vi "Generate Log Data.vi"(8 "error in (no error)":errorcluster, 11 "TestRec":T1) -> (0 "error out":errorcluster, 3 "Log Data":string[][](array[string]), 5 "CsvPath":path)   [LabVIEW 2011]
uses:
  Controls/DVR of CSV Tests Data.ctl
  Controls/CSVs Tests Data.ctl
  Controls/Test Column Data.ctl
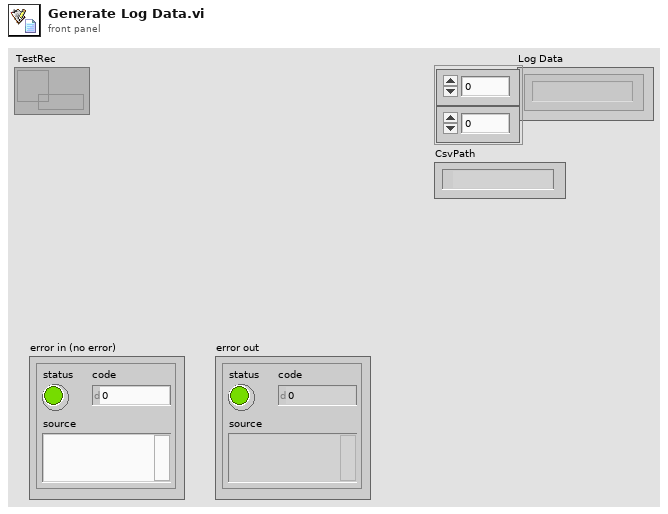
[diagram p1: front panel]
types:
  T1 = typedef "DVR of CSV Tests Data.ctl" = refnum<data-value>
  T2 = typedef "CSVs Tests Data.ctl" = cluster{"Test Data":T3[], "CsvPath":path, "LogPath":path, "Pass?":bool, "Error":errorcluster}
  T3 = typedef "Test Column Data.ctl" = cluster{"Chn":string, "ExpVals":dbl[], "TimeStamps":i64[], "NegTol":dbl, "PosTol":dbl}
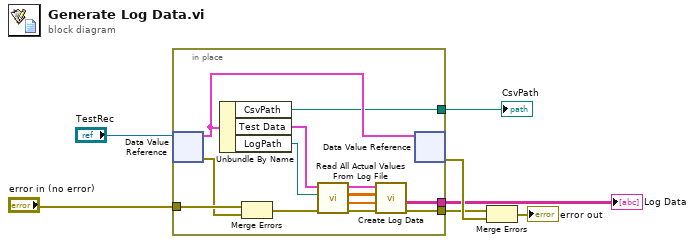
[diagram p0: block diagram]
diagram:
  n1 = in-place {
    in-place-border: "error in (no error)" -> [w20]
    in-place-border: [w10] -> w3
    in-place-border: [w9] -> w2
    in-place-border: [w8] -> w1
    n2 = in-place-dvr #1("TestRec") -> (w18:T2, w19:errorcluster)
    n3 = Unbundle By Name(w18) -> ("CsvPath"=w8:path, "Test Data"=w16:T3[], "LogPath"=w15:path)
    n4 = Merge Errors(w20, w19) -> (w17:errorcluster)
    n5 = call "Read All Actual Values From Log File.vi"("Error In"=w17, "Log"=w15, "Test Data"=w16) -> ("Error Out"=w11:errorcluster, "System Time"=w12:dbl[], "Actual Values"=w13:dbl[][], "Test Data dup"=w14:T3[])  [unwired: 5 in]
    n6 = call "Create Log Data.vi"("error in (no error)"=w11, "System Time"=w12, "Actual Values"=w13, "Test Data"=w14) -> ("error out"=w10:errorcluster, "Log Data"=w9:string[][])  [unwired: 6 in]
    n7 = in-place-dvr #1(w18) -> (w6:errorcluster)  [unwired: 1 out]
  }
  "Log Data" <- w2
  "CsvPath" <- w1
  n8 = Merge Errors(w3, w6) -> (→"error out":errorcluster)
